vi "Data_Aquisition_cRIO5.vi"() -> ()   [LabVIEW 2016]
uses:
  <vilib>/Platform/TimedLoop/XDataNode/timing_clust.ctl
  <vilib>/Platform/TimedLoop/XDataNode/nitl_modes.ctl
  <vilib>/Platform/TimedLoop/XDataNode/wakeup.ctl
  <vilib>/Utility/file.llb/Write Delimited Spreadsheet (string).vi
  <vilib>/Platform/TimedLoop/XDataNode/loadnilvce.vi
  <vilib>/Utility/file.llb/Write Delimited Spreadsheet (DBL).vi
  <vilib>/Platform/TimedLoop/XDataNode/XDataNode.xnode
  <vilib>/Platform/TimedLoop/XDataNode/XDNodeRunTimeDep.lvlib
panel:
  out "Data":dbl[][](array[numeric])
  out "Headers":string[][](array[string])
  in  "Mod 3 Labels":string[][](array[string])
  in  "Mod 2 Labels":string[][](array[string])
  in  "Mod 1 Labels":string[][](array[string])
  out "Time":string="123826.71"
  out "Date":string="04162018"
  in  "Buffer Size":i32=100
  out "Saving?":bool=TRUE
  out "new file path (Not A Path if cancelled)":path=path "u:/_04162018_123759.csv"
  in  "File Name:":string
  out "error out":errorcluster
  out "iter number":i32=2717
  in  "stop":bool
  in  "error in":errorcluster
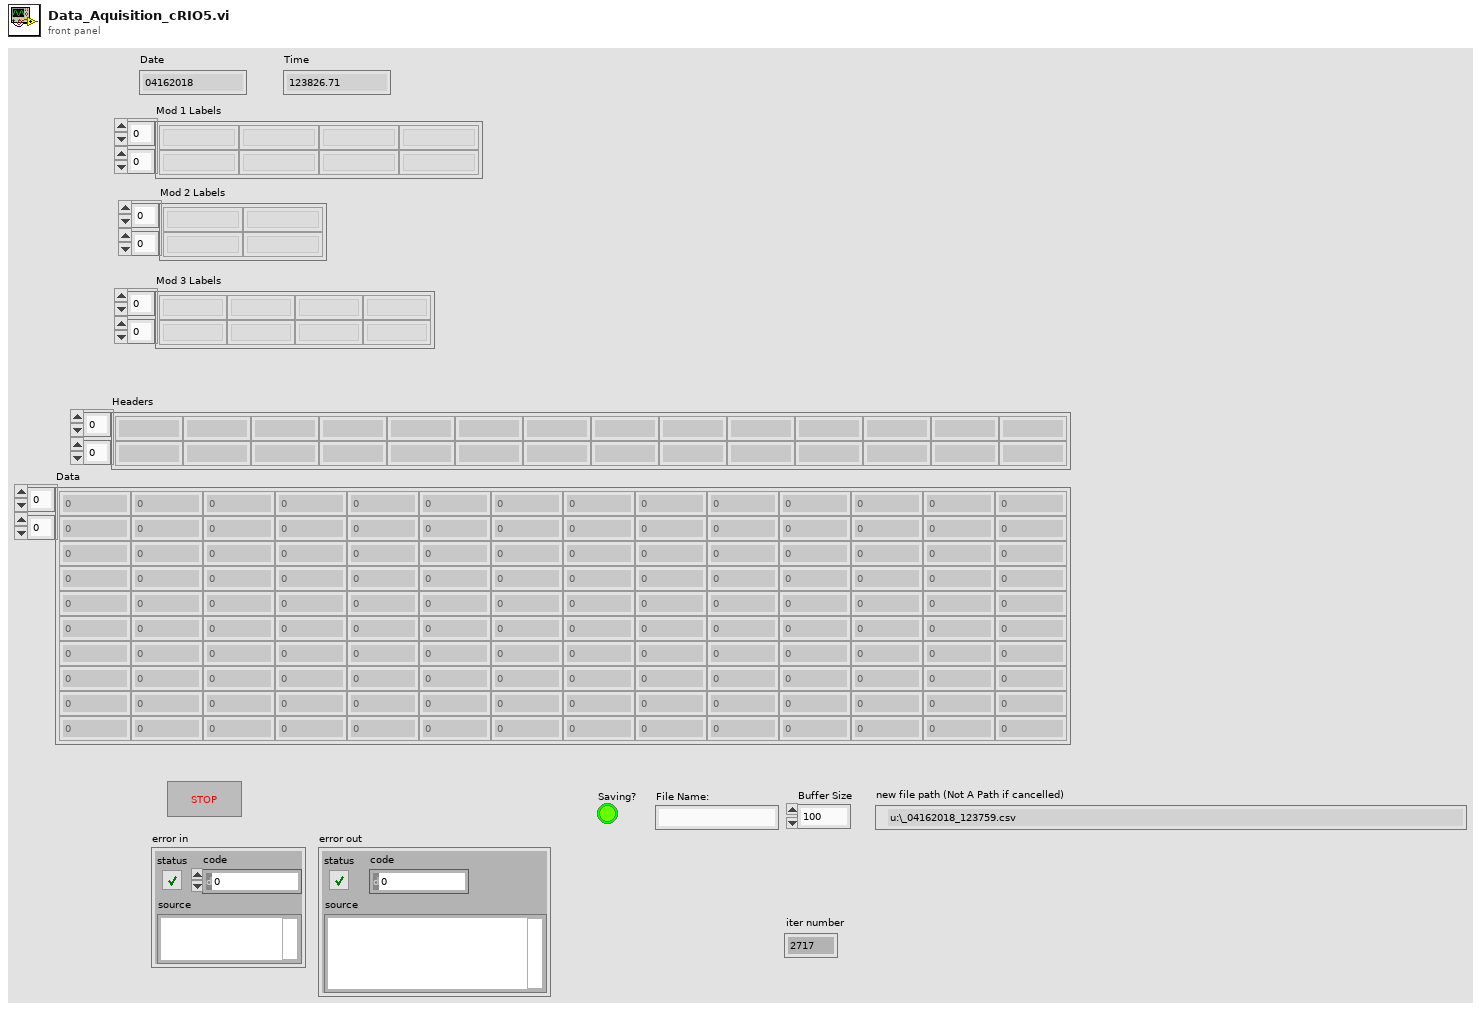
[diagram p1: front panel]
types:
  T1 = typedef "XDNodeRunTimeDep.lvlib/timing_clust.ctl" = cluster{"Expected End [f-1]":u64, "Actual End [f-1]":u64, "Finished Late? [f-1]":bool, "Expected End [i-1]":u64, "Actual End [i-1]":u64, "Finished Late? [i-1]":bool, "Expected Start [i]":u64, "Actual Start [i]":u64, "Expected Start [f]":u64, "Actual Start [f]":u64, "Source Name":string, "Structure Name":string, "Period":i64, "Deadline":i64, "Offset":i64, "Start":i64, "Priority":i32, "Timeout":i32, "Mode":T2, "Wakeup Reason":T3, "Error":errorcluster, "Source Type":string, "Secondary Source Type":string, "Global End Time":u64, "Global Start Time":u64, "Frame Duration":u64, "Iteration Duration":u64, "Assigned CPU":i32, "I/O Scan Engine Mode":u32}
  T2 = typedef "XDNodeRunTimeDep.lvlib/nitl_modes.ctl" = enum32{"No Change", "Process missed periods, maintain original phase", "Discard missed periods, maintain original phase", "Process missed periods, ignore original phase", "Discard missed periods, ignore original phase"}
  T3 = typedef "XDNodeRunTimeDep.lvlib/wakeup.ctl" = enum32{"Normal", "Aborted", "Asynchronous wakeup", "Timing source error", "Timed loop error", "Timeout"}
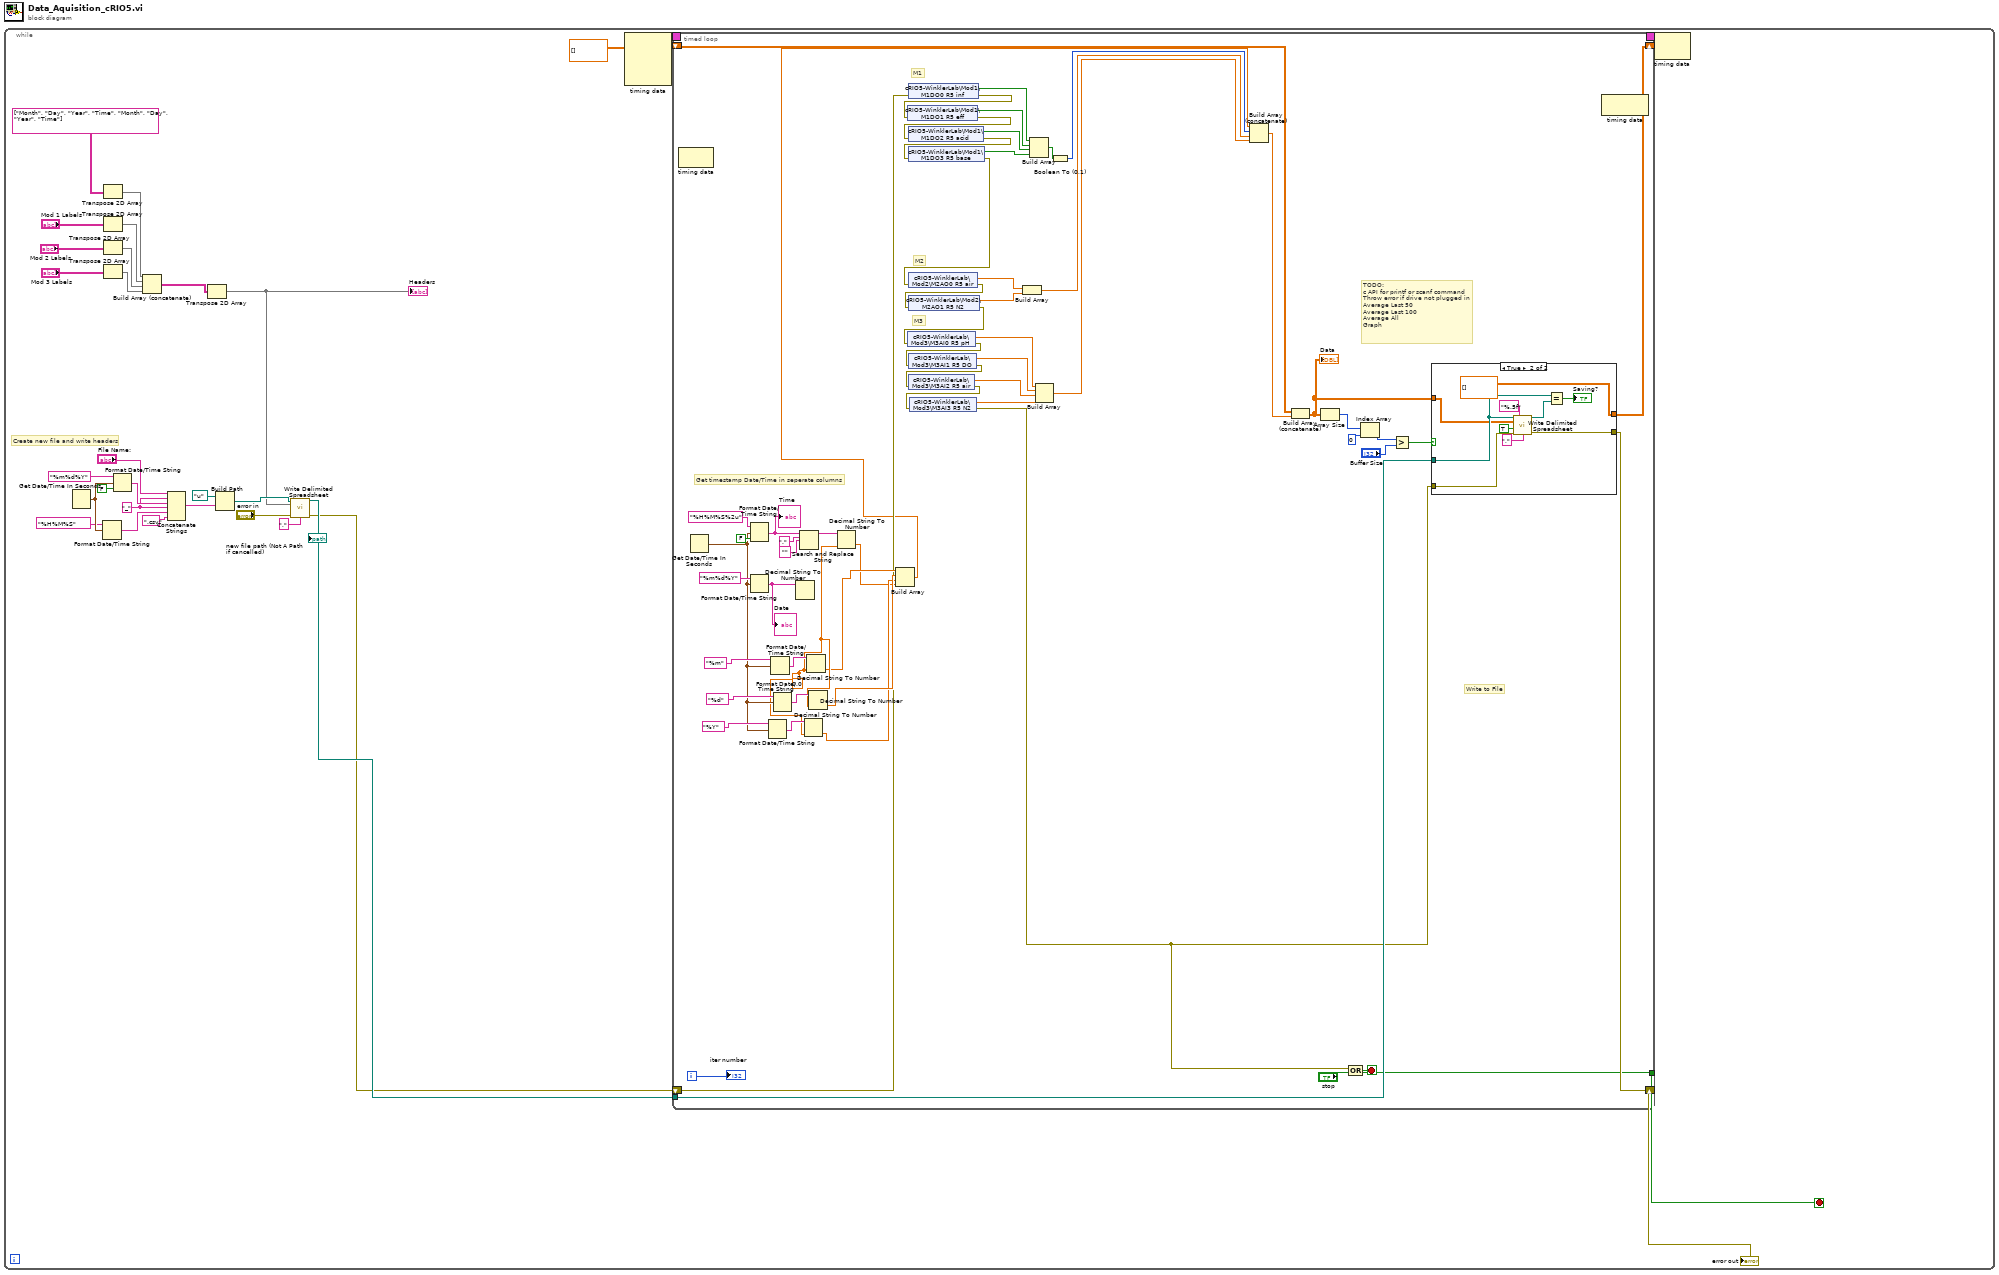
[diagram p0: block diagram]
diagram:
  n1 = while {
    stop <- w16 stop-if-true
    w19 = "_" ("string")
    # "Create new file and write headers"
    n2 = Get Date/Time In Seconds() -> (seconds since 1Jan1904=w24:timestamp)
    n3 = Format Date/Time String(time format string (%c)="%H%M%S", seconds (now)=w24) -> (date/time string=w18:string)  [unwired: 1 in]
    n4 = Transpose 2D Array(2D array=string[][] [["Month", "Day", "Year", "Time"], ["Month", "Day", "Year", "Time"]]) -> (transposed array=w8:string[][])
    n5 = Transpose 2D Array(2D array="Mod 1 Labels") -> (transposed array=w7:string[][])
    n6 = Transpose 2D Array(2D array="Mod 2 Labels") -> (transposed array=w6:string[][])
    n7 = Transpose 2D Array(2D array="Mod 3 Labels") -> (transposed array=w5:string[][])
    n8 = Format Date/Time String(time format string (%c)="%m%d%Y", seconds (now)=w24, UTC format=FALSE) -> (date/time string=w20:string)
    n9 = Build Array (concatenate)(w8, w7, w6, w5) -> (w10:string[][])
    n10 = Concatenate Strings("File Name:", w19, w20, w19, w18, ".csv" ("string")) -> (w17:string)
    n11 = Transpose 2D Array(2D array=w10) -> (transposed array=w1:string[][])
    "Headers" <- w1
    n12 = Build Path(base path=path "u:/" ("Save to:"), name or relative path=w17) -> (appended path=w27:path)
    n13 = call-poly <vilib>:"Write Delimited Spreadsheet.vi"("file path (dialog if empty)"=w27, "2D data"=w1, "error in (no error)"="error in", "delimiter (\\t)"="," ("delimiter (\\t)")) -> ("new file path (Not A Path if cancelled)"=w31:path, "error out"=w30:errorcluster)  [unwired: 10 in]
    "new file path (Not A Path if cancelled)" <- w31
    n14 = node-c288() -> (w15:T1)  [unwired: 4 in]
    n15 = timed-loop {
      tunnel: w31 -> [w84]
      shift-right: [w70] -> _
      shift-left: dbl[][] [] -> [w89]
      shift-right: [w82] -> w11
      shift-left: w30 -> [w54]
      tunnel: ["stop"] -> w16
      timing: w15 -> [_]
      timing-out: [_] -> w14
      i -> [w90]
      stop <- w91 stop-if-true
      w62 = 0.0
      # "M3"
      # "M2"
      # "M1"
      # "TODO: \nc API for printf or scanf command\nThrow error if drive not plugged in\nAverage Last 50\nAverage Last 100\nAverage All\nGraph"
      # "Write to File"
      # "Get timestamp Date/Time in seperate columns"
      n16 = node-c288() -> ()  [unwired: 1 in, 1 out]
      n17 = Get Date/Time In Seconds() -> (seconds since 1Jan1904=w63:timestamp)
      n18 = Format Date/Time String(time format string (%c)="%H%M%S%2u", seconds (now)=w63, UTC format=FALSE) -> (date/time string=w77:string)
      "Time" <- w77
      n19 = Format Date/Time String(time format string (%c)="%m%d%Y", seconds (now)=w63) -> (date/time string=w74:string)  [unwired: 1 in]
      "Date" <- w74
      n20 = Format Date/Time String(time format string (%c)="%Y", seconds (now)=w63) -> (date/time string=w64:string)  [unwired: 1 in]
      n21 = Format Date/Time String(time format string (%c)="%m", seconds (now)=w63) -> (date/time string=w68:string)  [unwired: 1 in]
      n22 = Format Date/Time String(time format string (%c)="%d", seconds (now)=w63) -> (date/time string=w66:string)  [unwired: 1 in]
      n23 = Decimal String To Number(string=w74) -> ()  [unwired: 2 in, 2 out]
      n24 = Search and Replace String(input string=w77, search string=".", replace string="") -> (result string=w76:string)  [unwired: 5 in, 3 out]
      n25 = Decimal String To Number(string=w64, default (0L)=w62) -> (number=w59:dbl)  [unwired: 1 in, 1 out]
      n26 = Decimal String To Number(string=w68, default (0L)=w62) -> (number=w61:dbl)  [unwired: 1 in, 1 out]
      n27 = Decimal String To Number(string=w66, default (0L)=w62) -> (number=w60:dbl)  [unwired: 1 in, 1 out]
      n28 = Decimal String To Number(string=w76, default (0L)=w62) -> (number=w58:dbl)  [unwired: 1 in, 1 out]
      n29 = Build Array(w61, w60, w59, w58) -> (w43:dbl[])
      n30 = shared-variable "cRIO5-WinklerLab\\Mod1\\M1DO0 R5 inf"(error in=w54) -> (w53:bool, error out=w57:errorcluster)
      n31 = shared-variable "cRIO5-WinklerLab\\Mod1\\M1DO1 R5 eff"(error in=w57) -> (w52:bool, error out=w56:errorcluster)
      n32 = shared-variable "cRIO5-WinklerLab\\Mod1\\M1DO2 R5 acid"(error in=w56) -> (w51:bool, error out=w55:errorcluster)
      n33 = shared-variable "cRIO5-WinklerLab\\Mod1\\M1DO3 R5 base"(error in=w55) -> (w50:bool, error out=w34:errorcluster)
      n34 = shared-variable "cRIO5-WinklerLab\\Mod2\\M2AO0 R5 air"(error in=w34) -> (w48:dbl, error out=w49:errorcluster)
      n35 = shared-variable "cRIO5-WinklerLab\\Mod2\\M2AO1 R5 N2"(error in=w49) -> (w47:dbl, error out=w39:errorcluster)
      n36 = shared-variable "cRIO5-WinklerLab\\Mod3\\M3AI0 R5 pH"(error in=w39) -> (w38:dbl, error out=w42:errorcluster)
      n37 = shared-variable "cRIO5-WinklerLab\\Mod3\\M3AI1 R5 DO"(error in=w42) -> (w37:dbl, error out=w41:errorcluster)
      n38 = shared-variable "cRIO5-WinklerLab\\Mod3\\M3AI2 R5 air"(error in=w41) -> (w36:dbl, error out=w40:errorcluster)
      n39 = shared-variable "cRIO5-WinklerLab\\Mod3\\M3AI3 R5 N2"(error in=w40) -> (w35:dbl, error out=w33:errorcluster)
      n40 = Build Array(w48, w47) -> (w45:dbl[])
      n41 = Build Array(w53, w52, w51, w50) -> (w46:bool[])
      n42 = Build Array(w38, w37, w36, w35) -> (w72:dbl[])
      n43 = Boolean To (0,1)(Boolean=w46) -> (0, 1=w44:i16[])
      n44 = Build Array (concatenate)(w43, w44, w45, w72) -> (w71:dbl[])
      n45 = Build Array (concatenate)(w89, w71) -> (w32:dbl[][])
      "Data" <- w32
      n46 = Array Size(array=w32) -> (size(s)=w88:i32[])
      n47 = Compound Arithmetic op=OR(w33, "stop") -> (w91:bool)
      n48 = Index Array(array=w88, index=0) -> (element=w86:i32)
      n49 = Greater?(x=w86, y="Buffer Size") -> (0:w85:bool)
      n50 = case shown="True" w85 {
        tunnel: w32 -> [w95 w96]
        tunnel: w84 -> [_ w103]
        tunnel: [w95 dbl[][] []] -> w70
        tunnel: [w94 w102] -> w82
        tunnel: w33 -> [w94 w97]
        frame False {
        }
        frame True {
          n51 = call-poly <vilib>:"Write Delimited Spreadsheet.vi"("file path (dialog if empty)"=w103, "format (%.3f)"="%.5f", "2D data"=w96, "append to file? (new file:F)"=TRUE, "error in (no error)"=w97, "delimiter (\\t)"="," ("delimiter (\\t)")) -> ("new file path (Not A Path if cancelled)"=w104:path, "error out"=w102:errorcluster)  [unwired: 8 in]
          n52 = Equal?(x=w103, y=w104) -> (x = y?=→"Saving?":bool)
        }
      }
      n53 = node-c288() -> ()  [unwired: 1 in, 1 out]
      "iter number" <- w90
    }
    "error out" <- w11
    n54 = node-c288(w14) -> ()  [unwired: 1 out]
  }
